vi "Background Process Directors.vi"(8 "error in (no error)":errorcluster, 10 "Wait Time":u32 caption="ms" step=1, 11 "TestProcessor in":refnum<class "TestProcessor.lvclass">) -> (0 "error out":errorcluster, 3 "TestProcessor out":refnum<class "TestProcessor.lvclass">)   [LabVIEW 2023, in "HAF.lvlib" / "TestProcessor.lvclass"]
doc: "Calls the Process Directors method asynchronously, without waiting for a result (Process Director notifies results.)  Using this approach means the User Test Application UI isn’t blocked by long-running Commands and can remain responsive to result notifications."
uses:
  TestProcessor.lvclass
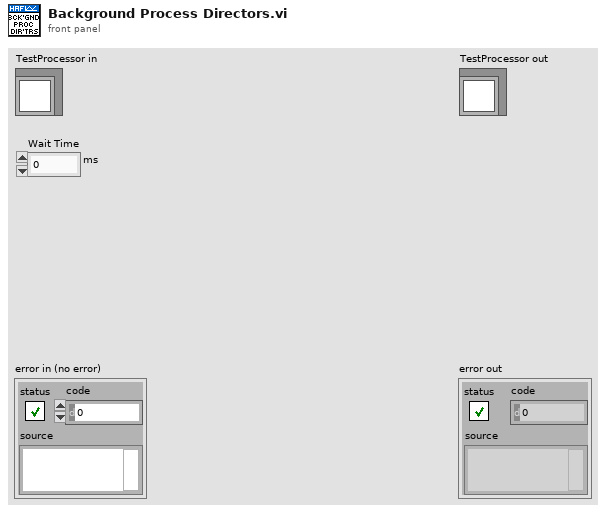
[diagram p1: front panel]
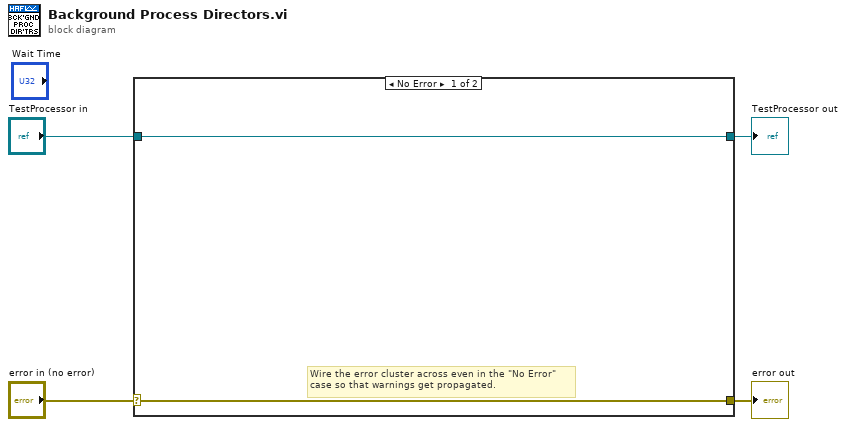
[diagram p0: block diagram]
diagram:
  n1 = case shown="No Error" "error in (no error)" {
    selector: "error in (no error)" -> [w5 w8]
    tunnel: [w5 w8] -> w3
    tunnel: [w6 w7] -> w1
    tunnel: "TestProcessor in" -> [w6 w7]
    frame No Error {
      # "Wire the error cluster across even in the \"No Error\"\ncase so that warnings get propagated."
    }
    frame Error {
    }
  }
  "error out" <- w3
  "TestProcessor out" <- w1
